vi "Power Maximizer.vi"() -> ()   [LabVIEW 2010]
uses:
  <vilib>/express/express analysis/Spectral/XNode/ExpressSpectralMeasurementsBlockNode.xnode
  <vilib>/express/express analysis/Spectral/Block/exnSpectralBlock spectral measurements RMS poly.vi
  <vilib>/express/express analysis/Spectral/Block/exnSpectralBlock spectral measurements RMS WFM.vi
  <vilib>/Analysis/NI_AALPro.lvlib
panel:
  out "slope":dbl
  out "intercept":dynamicdata(graph)
  out "mean squared error":dynamicdata(graph)
  out "residual":dynamicdata(graph)
  out "Rxx":dynamicdata(graph)
  in  "Minimum Threshold":dbl=6e-05 format="%.3p"
  out "Actual Power":dbl format="%.3p"
  out "Power below Treshold":bool
  in  "Thin Etalon Position Setpoint":dbl
  in  "Correction Threshold":dbl=2e-06 format="%.3p"
  out "Maximum Power (Window)":dbl format="%#.3p"
  out "best fit 2":dbl
  out "best fit":dynamicdata(graph)
  out "falling":bool
  out "rising":bool
  out "size(s)":i32
  in  "Statistic Values Limit":i32=3600
  out "NB-TiSa Power vs Time":cluster{cluster{dbl, "Value":dbl}[]}[](graph)
  in  "Max Values Limit":i32=3600
  out "New Power Value":bool
  in  "stop":bool
  out "loop counter":i32
  out "MPM Ch7 Reference Power":dbl format="%.3p"
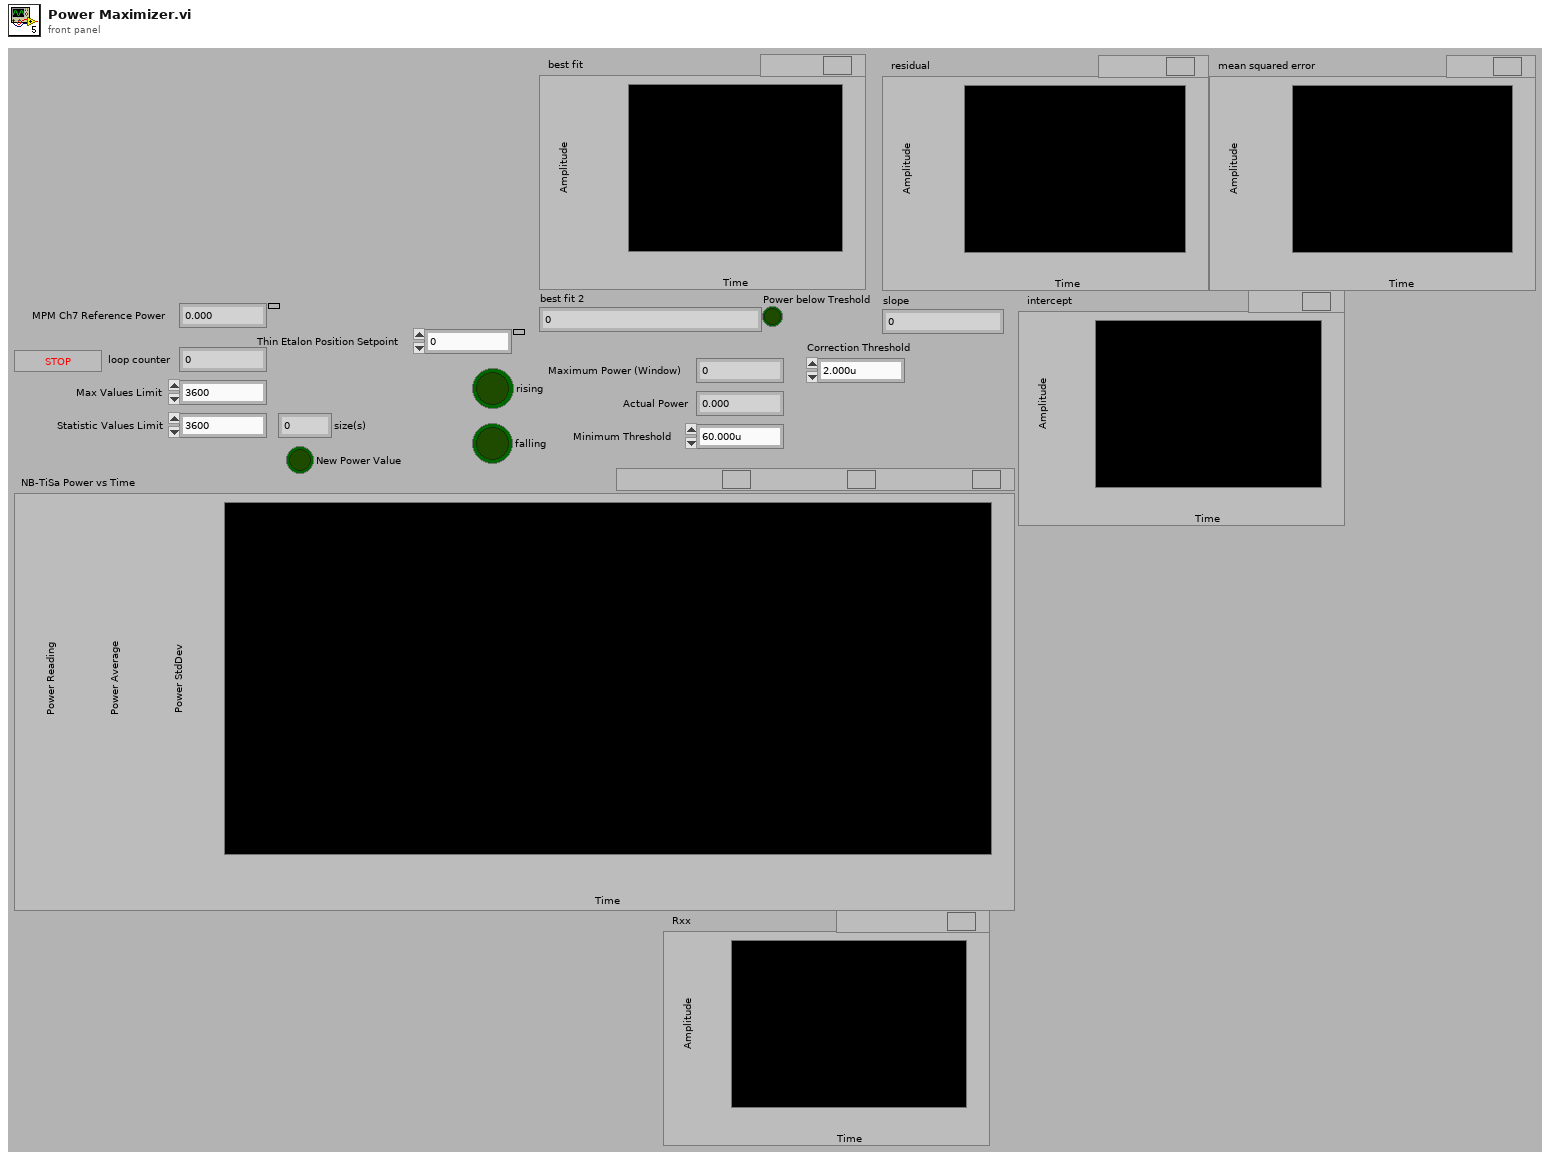
[diagram p1: front panel]
types:
  T1 = cluster{"averaging mode":u16, "weighting mode":u16, "number of averages":u32}
  T2 = cluster{"dB On (F)":bool, "unwrap phase (F)":bool, "convert to degree (F)":bool}
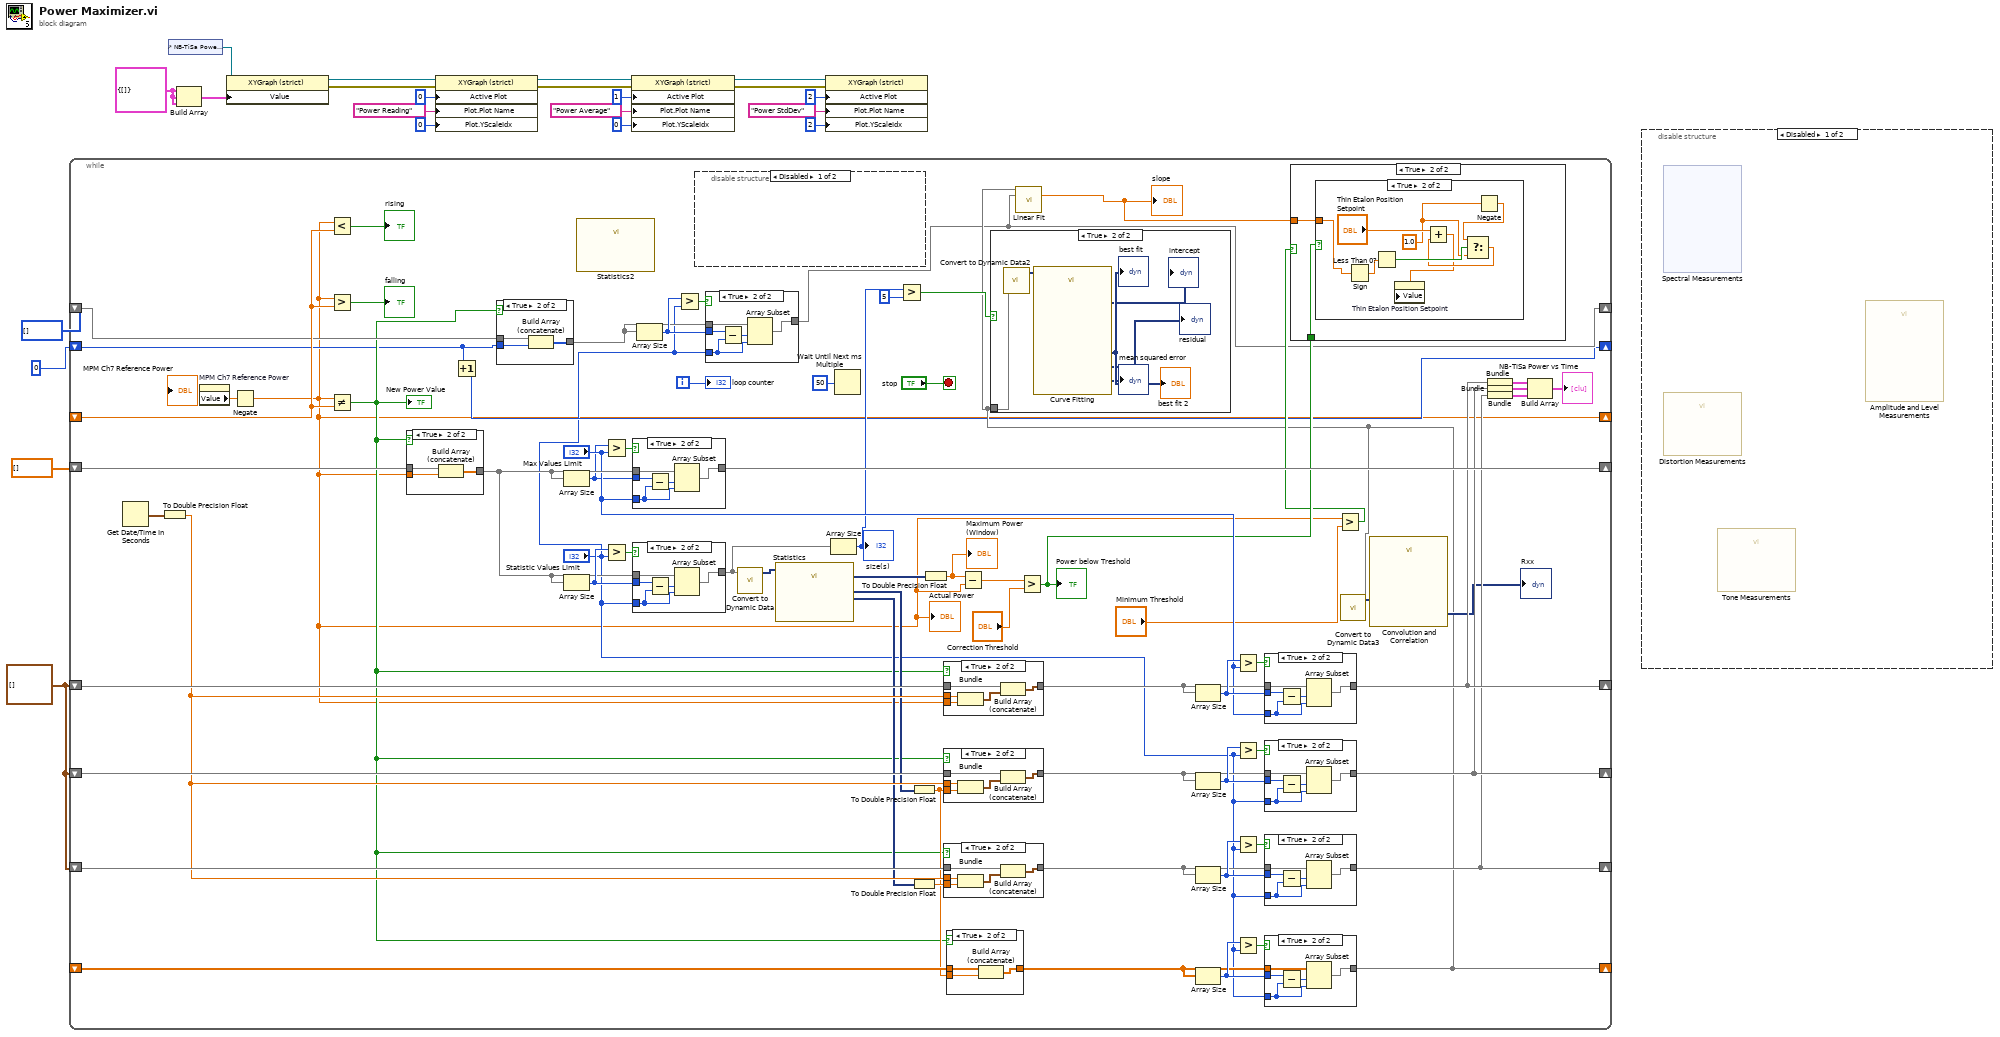
[diagram p0: block diagram]
diagram:
  w3 = cluster{dbl, dbl}[] []
  w10 = cluster{cluster{dbl, "Value":dbl}[]} {[]} ("output cluster")
  n1 = while {
    shift-right: [w23] -> _
    shift-left: _ -> [w57]
    shift-right: [w89] -> _
    shift-left: dbl[] [] -> [w90]
    shift-right: [w61] -> _
    shift-left: w3 -> [w76]
    shift-right: [w59] -> _
    shift-left: w3 -> [w75]
    shift-right: [w67] -> _
    shift-left: w3 -> [w77]
    shift-right: [w36] -> _
    shift-left: _ -> [w38]
    shift-right: [w29] -> _
    shift-left: i32[] [] -> [w33]
    shift-right: [w26] -> _
    shift-left: 0 -> [w27]
    i -> [w31]
    stop <- "stop" stop-if-true
    n2 = Get Date/Time In Seconds() -> (seconds since 1Jan1904=w87:timestamp)
    n3 = To Double Precision Float(number=w87) -> (double precision float=w74:dbl)
    n4 = property on="MPM Ch7 Reference Power" class="DigNum (strict)"() -> ("Value"=w91:dbl)  [unwired: 2 in, 2 out]
    n5 = Negate(x=w91) -> (-x=w23:dbl)
    "Actual Power" <- w23
    n6 = Less?(x=w23, y=w57) -> (x < y?=→"rising":bool)
    n7 = Greater?(x=w23, y=w57) -> (0:→"falling":bool)
    n8 = Not Equal?(x=w23, y=w57) -> (x != y?=w30:bool)
    "New Power Value" <- w30
    n9 = case shown="True" w30 {
      tunnel: [w177 w180] -> w79
      tunnel: w90 -> [w177 w179]
      tunnel: w23 -> [_ w178]
      frame False {
      }
      frame True {
        n10 = Build Array (concatenate)(w179, w178) -> (w180:dbl[])
      }
    }
    n11 = Increment(x=w27) -> (x+1=w26:i32)
    n12 = case shown="True" w30 {
      tunnel: [w99 w102] -> w32
      tunnel: w33 -> [w99 w101]
      tunnel: w27 -> [_ w100]
      frame False {
      }
      frame True {
        n13 = Build Array (concatenate)(w101, w100) -> (w102:i32[])
      }
    }
    n14 = Array Size(array=w79) -> (size(s)=w28:i32)
    n15 = Array Size(array=w79) -> (size(s)=w81:i32)
    n16 = call "Statistics2"() -> ()  [unwired: 27 in, 1 out]
    n17 = Greater?(x=w28, y="Max Values Limit") -> (0:w86:bool)
    n18 = Greater?(x=w81, y="Statistic Values Limit") -> (0:w80:bool)
    n19 = case shown="True" w86 {
      tunnel: w79 -> [w171 w175]
      tunnel: [w171 w174] -> w89
      tunnel: w28 -> [_ w173]
      tunnel: "Max Values Limit" -> [_ w172]
      frame False {
      }
      frame True {
        n20 = Subtract(x=w173, y=w172) -> (x-y=w176:i32)
        n21 = Array Subset(array=w175, index=w176, length=w172) -> (w174:dbl[])
      }
    }
    n22 = case shown="True" w80 {
      tunnel: w79 -> [w165 w169]
      tunnel: [w165 w168] -> w44
      tunnel: w81 -> [_ w167]
      tunnel: "Statistic Values Limit" -> [_ w166]
      frame False {
      }
      frame True {
        n23 = Subtract(x=w167, y=w166) -> (x-y=w170:i32)
        n24 = Array Subset(array=w169, index=w170, length=w166) -> (w168:dbl[])
      }
    }
    n25 = Array Size(array=w32) -> (size(s)=w35:i32)
    n26 = Greater?(x=w35, y="Statistic Values Limit") -> (0:w34:bool)
    n27 = disable-structure shown="Disabled" {
      frame Disabled {
      }
      frame Enabled {
      }
    }
    n28 = case shown="True" w34 {
      tunnel: w32 -> [w93 w97]
      tunnel: [w93 w96] -> w29
      tunnel: w35 -> [_ w95]
      tunnel: "Statistic Values Limit" -> [_ w94]
      frame False {
      }
      frame True {
        n29 = Subtract(x=w95, y=w94) -> (x-y=w98:i32)
        n30 = Array Subset(array=w97, index=w98, length=w94) -> (w96:i32[])
      }
    }
    n31 = call "Convert to Dynamic Data"("Array"=w44) -> ("Dynamic Data Type"=w78:dynamicdata)  [unwired: 3 in]
    n32 = call "Statistics"("Signals"=w78) -> ("Standard Dev"=w71:dynamicdata, "Arithmetic Mean"=w72:dynamicdata, "Maximum"=w51:dynamicdata)  [unwired: 22 in, 2 out]
    n33 = Array Size(array=w44) -> (size(s)=w54:i32)
    "size(s)" <- w54
    n34 = Wait Until Next ms Multiple(millisecond multiple=u32 50) -> ()  [unwired: 1 out]
    n35 = Greater?(x=w54, y=5) -> (0:w52:bool)
    n36 = To Double Precision Float(number=w72) -> (double precision float=w37:dbl)
    n37 = To Double Precision Float(number=w71) -> (double precision float=w73:dbl)
    n38 = To Double Precision Float(number=w51) -> (double precision float=w49:dbl)
    "Maximum Power (Window)" <- w49
    n39 = case shown="True" w30 {
      tunnel: [w159 w164] -> w68
      tunnel: w77 -> [w159 w163]
      tunnel: w23 -> [_ w161]
      tunnel: w74 -> [_ w162]
      frame False {
      }
      frame True {
        n40 = Bundle(w162, w161) -> (w160:cluster{dbl, dbl})  [unwired: 1 in]
        n41 = Build Array (concatenate)(w163, w160) -> (w164:cluster{dbl, dbl}[])
      }
    }
    n42 = case shown="True" w30 {
      tunnel: [w153 w158] -> w62
      tunnel: w76 -> [w153 w157]
      tunnel: w37 -> [_ w155]
      tunnel: w74 -> [_ w156]
      frame False {
      }
      frame True {
        n43 = Bundle(w156, w155) -> (w154:cluster{dbl, dbl})  [unwired: 1 in]
        n44 = Build Array (concatenate)(w157, w154) -> (w158:cluster{dbl, dbl}[])
      }
    }
    n45 = case shown="True" w30 {
      tunnel: [w147 w152] -> w60
      tunnel: w75 -> [w147 w151]
      tunnel: w73 -> [_ w149]
      tunnel: w74 -> [_ w150]
      frame False {
      }
      frame True {
        n46 = Bundle(w150, w149) -> (w148:cluster{dbl, dbl})  [unwired: 1 in]
        n47 = Build Array (concatenate)(w151, w148) -> (w152:cluster{dbl, dbl}[])
      }
    }
    n48 = case shown="True" w30 {
      tunnel: [w109 w112] -> w39
      tunnel: w38 -> [w109 w111]
      tunnel: w37 -> [_ w110]
      frame False {
      }
      frame True {
        n49 = Build Array (concatenate)(w111, w110) -> (w112:dbl[])
      }
    }
    n50 = Subtract(x=w49, y=w23) -> (x-y=w46:dbl)
    n51 = Greater?(x=w46, y="Correction Threshold") -> (0:w48:bool)
    "Power below Treshold" <- w48
    n52 = Array Size(array=w68) -> (size(s)=w70:i32)
    n53 = Array Size(array=w62) -> (size(s)=w65:i32)
    n54 = Array Size(array=w60) -> (size(s)=w64:i32)
    n55 = Array Size(array=w39) -> (size(s)=w40:i32)
    n56 = Greater?(x=w70, y="Max Values Limit") -> (0:w69:bool)
    n57 = Greater?(x=w65, y="Statistic Values Limit") -> (0:w66:bool)
    n58 = Greater?(x=w64, y="Statistic Values Limit") -> (0:w63:bool)
    n59 = Greater?(x=w40, y="Statistic Values Limit") -> (0:w41:bool)
    n60 = case shown="True" w69 {
      tunnel: w68 -> [w141 w145]
      tunnel: [w141 w144] -> w67
      tunnel: w70 -> [_ w143]
      tunnel: "Max Values Limit" -> [_ w142]
      frame False {
      }
      frame True {
        n61 = Subtract(x=w143, y=w142) -> (x-y=w146:i32)
        n62 = Array Subset(array=w145, index=w146, length=w142) -> (w144:cluster{dbl, dbl}[])
      }
    }
    n63 = case shown="True" w66 {
      tunnel: w62 -> [w135 w139]
      tunnel: [w135 w138] -> w61
      tunnel: w65 -> [_ w137]
      tunnel: "Statistic Values Limit" -> [_ w136]
      frame False {
      }
      frame True {
        n64 = Subtract(x=w137, y=w136) -> (x-y=w140:i32)
        n65 = Array Subset(array=w139, index=w140, length=w136) -> (w138:cluster{dbl, dbl}[])
      }
    }
    n66 = case shown="True" w63 {
      tunnel: w60 -> [w129 w133]
      tunnel: [w129 w132] -> w59
      tunnel: w64 -> [_ w131]
      tunnel: "Statistic Values Limit" -> [_ w130]
      frame False {
      }
      frame True {
        n67 = Subtract(x=w131, y=w130) -> (x-y=w134:i32)
        n68 = Array Subset(array=w133, index=w134, length=w130) -> (w132:cluster{dbl, dbl}[])
      }
    }
    n69 = case shown="True" w41 {
      tunnel: w39 -> [w103 w107]
      tunnel: [w103 w106] -> w36
      tunnel: w40 -> [_ w105]
      tunnel: "Statistic Values Limit" -> [_ w104]
      frame False {
      }
      frame True {
        n70 = Subtract(x=w105, y=w104) -> (x-y=w108:i32)
        n71 = Array Subset(array=w107, index=w108, length=w104) -> (w106:dbl[])
      }
    }
    n72 = case shown="True" w52 {
      tunnel: w36 -> [_ w128]
      frame False {
      }
      frame True {
        n73 = call "Convert to Dynamic Data2"("Array"=w128) -> ("Dynamic Data Type"=w127:dynamicdata)  [unwired: 3 in]
        n74 = call "Curve Fitting"("Signals"=w127) -> ("mean squared error"=→"mean squared error":dynamicdata, "residual"=→"residual":dynamicdata, "best fit"=→"best fit" →"best fit 2":dynamicdata, "intercept"=→"intercept":dynamicdata)  [unwired: 6 in, 1 out]
      }
    }
    n75 = call <vilib>:"Linear Fit.vi"("Y"=w36, "X"=w29) -> ("slope"=w24:dbl)  [unwired: 9 in, 4 out]
    "slope" <- w24
    n76 = Greater?(x=w23, y="Minimum Threshold") -> (0:w45:bool)
    n77 = case shown="True" w45 {
      tunnel: w48 -> [_ w114]
      tunnel: w24 -> [_ w113]
      frame False {
      }
      frame True {
        n78 = case shown="True" w114 {
          tunnel: w113 -> [_ w122]
          frame False {
          }
          frame True {
            w115 = 1.0 ("y")
            n79 = Sign(1:w122) -> (0:w121:dbl)
            n80 = Less Than 0?(x=w121) -> (x < 0?=w119:bool)
            n81 = Negate(x=w115) -> (-x=w118:dbl)
            n82 = Select(t=w118, s=w119, f=w115) -> (s? t:f=w117:dbl)
            n83 = Add(x="Thin Etalon Position Setpoint", y=w117) -> (x+y=w116:dbl)
            n84 = property on="Thin Etalon Position Setpoint" class="DigNum (strict)"("Value"=w116) -> ()  [unwired: 2 in, 2 out]
          }
        }
      }
    }
    n85 = call "Convert to Dynamic Data3"("Array"=w36) -> ("Dynamic Data Type"=w43:dynamicdata)  [unwired: 3 in]
    n86 = call "Convolution and Correlation"("X"=w43) -> ("Rxx"=→"Rxx":dynamicdata)  [unwired: 9 in, 1 out]
    n87 = Bundle(w67) -> (w85:cluster{cluster{dbl, dbl}[]})  [unwired: 1 in]
    n88 = Bundle(w61) -> (w84:cluster{cluster{dbl, dbl}[]})  [unwired: 1 in]
    n89 = Bundle(w59) -> (w83:cluster{cluster{dbl, dbl}[]})  [unwired: 1 in]
    n90 = Build Array(w85, w84, w83) -> (→"NB-TiSa Power vs Time":cluster{cluster{dbl, dbl}[]}[])
    "loop counter" <- w31
  }
  n91 = control-ref of="NB-TiSa Power vs Time"() -> (w8:refnum<vi>)
  n92 = Build Array(w10, w10, w10) -> (w9:cluster{cluster{dbl, "Value":dbl}[]}[])
  n93 = property on="Property Node" class="XYGraph (strict)"(reference=w8, "Value"=w9) -> (reference out=w7:refnum<vi>, error out=w11:errorcluster)  [unwired: 1 in]
  n94 = property on="Property Node" class="XYGraph (strict)"(reference=w7, error in=w11, "Active Plot"=u32 0, "Plot.Plot Name"="Power Reading", "Plot.YScaleIdx"=u32 0 ("Plot.Y Scale Index")) -> (reference out=w6:refnum<vi>, error out=w21:errorcluster)
  n95 = property on="Property Node" class="XYGraph (strict)"(reference=w6, error in=w21, "Active Plot"=u32 1, "Plot.Plot Name"="Power Average", "Plot.YScaleIdx"=u32 0 ("Plot.Y Scale Index")) -> (reference out=w5:refnum<vi>, error out=w22:errorcluster)
  n96 = property on="Property Node" class="XYGraph (strict)"(reference=w5, error in=w22, "Active Plot"=u32 2, "Plot.Plot Name"="Power StdDev", "Plot.YScaleIdx"=u32 2 ("Plot.Y Scale Index")) -> ()  [unwired: 2 out]
  n97 = disable-structure shown="Disabled" {
    frame Disabled {
      n98 = xnode "Spectral Measurements"() -> ()  [unwired: 2 in, 3 out]
      n99 = call "Distortion Measurements"() -> ()  [unwired: 11 in, 1 out]
      n100 = call "Tone Measurements"() -> ()  [unwired: 8 in, 4 out]
      n101 = call "Amplitude and Level Measurements"() -> ()  [unwired: 14 in, 2 out]
    }
    frame Enabled {
    }
  }
